vi "Aerotech abort.vi"(8 "error in (no error)":errorcluster, 11 "AerotechStage in":refnum<class "AerotechStage.lvclass">) -> (0 "error out":errorcluster, 3 "AerotechStage out":refnum<class "AerotechStage.lvclass">)   [LabVIEW 2020, in "AerotechStage.lvclass"]
uses:
  AerotechStage.lvclass
  AerotechStage.lvclass/AerotechStage.ctl
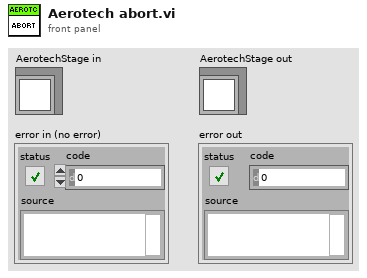
[diagram p1: front panel]
types:
  T1 = typedef "OnOffTypeDef.ctl" = enum16{"off", "on"}
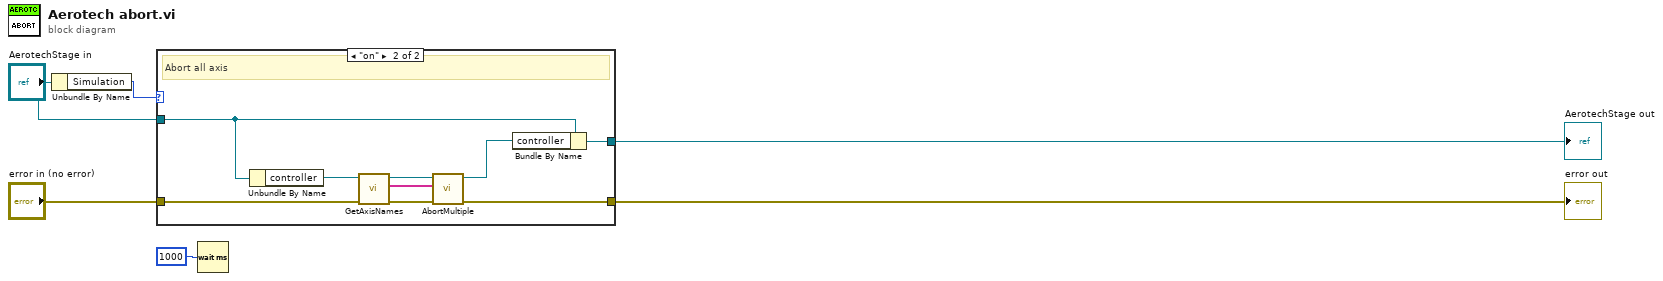
[diagram p0: block diagram]
diagram:
  n1 = Unbundle By Name("AerotechStage in") -> ("Simulation"=w2:T1)
  n2 = case shown="\"on\"" w2 {
    tunnel: "error in (no error)" -> [w7 w17]
    tunnel: "AerotechStage in" -> [w8 w12]
    tunnel: [w7 w10] -> w6
    tunnel: [w8 w9] -> w5
    frame "off", Default {
    }
    frame "on" {
      # "Abort all axis"
      n3 = Unbundle By Name(w12) -> ("controller"=w13:refnum<k24>)
      n4 = call "GetAxisNames.vi"("error in (no error)"=w17, "controller in"=w13) -> ("error out"=w16:errorcluster, "axis names"=w15:string[], "controller out"=w14:refnum<k24>)  [unwired: 7 in]
      n5 = call "AbortMultiple.vi"("error in (no error)"=w16, "axis names"=w15, "controller in"=w14) -> ("error out"=w10:errorcluster, "controller out"=w11:refnum<k24>)  [unwired: 7 in]
      n6 = Bundle By Name(cluster=w12, "controller"=w11) -> (w9:refnum<class "AerotechStage.lvclass">)
    }
  }
  "error out" <- w6
  "AerotechStage out" <- w5
  n7 = Wait (ms)(milliseconds to wait=u32 1000) -> ()  [unwired: 1 out]
